vi "checkandcreatefoldersforfullpath.vi"(4 "Path IN":path) -> (1 "Path OUT":path)   [LabVIEW 2012]
doc: "SciScan 1.2 160622"
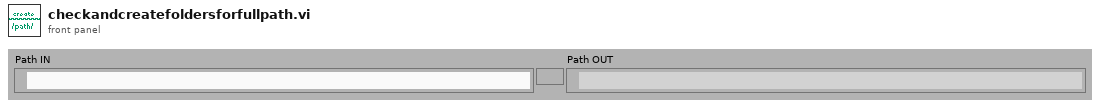
[diagram p1: front panel]
types:
  T1 = enum16{"open", "replace", "create", "open or create", "replace or create", "replace or create with confirmation"}
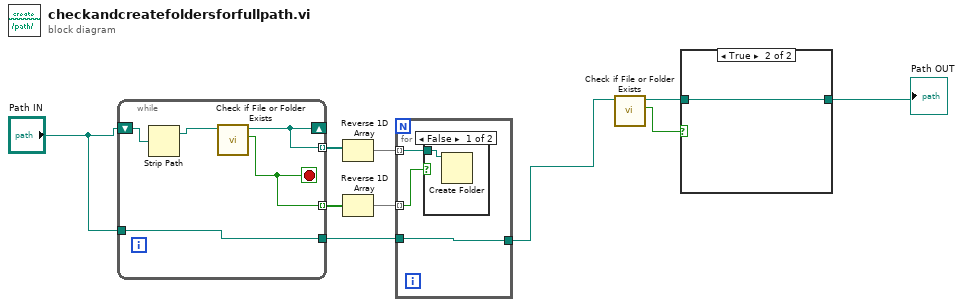
[diagram p0: block diagram]
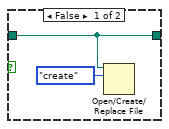
[diagram p2: hidden frame]
diagram:
  n1 = while {
    shift-right: [w13] -> _
    shift-left: "Path IN" -> [w14]
    tunnel: [w13] -> w10 mode=indexing
    tunnel: [w12] -> w8
    tunnel: "Path IN" -> [w12]
    tunnel: [w11] -> w7 mode=indexing
    stop <- w11 stop-if-true
    n2 = Strip Path(path=w14) -> (stripped path=w15:path)  [unwired: 1 out]
    n3 = call <vilib>:"Check if File or Folder Exists.vi"("path"=w15) -> ("file or folder exists?"=w11:bool, "dup path"=w13:path)  [unwired: 8 in, 1 out]
  }
  n4 = Reverse 1D Array(array=w10) -> (reversed array=w9:path[])
  n5 = Reverse 1D Array(array=w7) -> (reversed array=w6:bool[])
  n6 = for {
    tunnel: w9 -> [w18] mode=indexing
    tunnel: [w17] -> w4
    tunnel: w8 -> [w17]
    tunnel: w6 -> [w16] mode=indexing
    n7 = case shown="False" w16 {
      tunnel: w18 -> [w19 _]
      frame False {
        n8 = Create Folder(path (use dialog)=w19) -> ()  [unwired: 2 in, 3 out]
      }
      frame True {
      }
    }
  }
  n9 = call <vilib>:"Check if File or Folder Exists.vi"("path"=w4) -> ("file or folder exists?"=w2:bool, "dup path"=w3:path)  [unwired: 8 in, 1 out]
  n10 = case shown="True" w2 {
    tunnel: w3 -> [w20 w22]
    tunnel: [w20 w22] -> w1
    frame False {
      n11 = Open/Create/Replace File(file path (use dialog)=w20, operation (0:open)=T1."create") -> ()  [unwired: 4 in, 3 out]
    }
    frame True {
    }
  }
  "Path OUT" <- w1
